vi "Create PublicEvents.vi"(5 "PublicEvents in":refnum<class "PublicEvents.lvclass">, 8 "error in (no error)":errorcluster, 11 "SMO":refnum<class "SMO.lvclass">) -> (0 "error out":errorcluster, 3 "PublicEvents":refnum<class "PublicEvents.lvclass">)   [LabVIEW 2013, in "PublicEvents.lvclass"]
uses:
  PublicEvents.lvclass
  SMO/SMO.lvclass
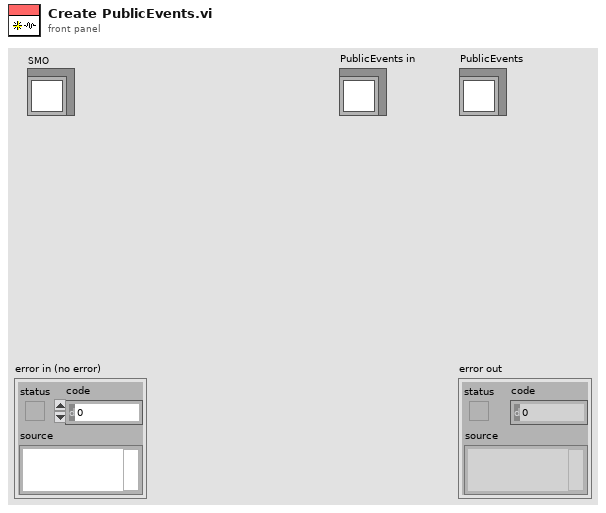
[diagram p1: front panel]
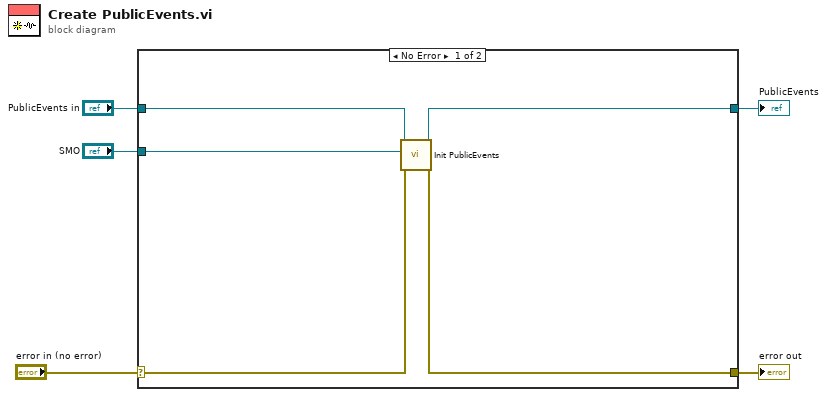
[diagram p0: block diagram]
diagram:
  n1 = case shown="No Error" "error in (no error)" {
    selector: "error in (no error)" -> [w8 w12]
    tunnel: [w7 w12] -> w4
    tunnel: [w9 w11] -> w3
    tunnel: "PublicEvents in" -> [w10 w11]
    tunnel: "SMO" -> [w6 _]
    frame No Error {
      n2 = call-dynamic "Init PublicEvents.vi"("error in (no error)"=w8, "SMO"=w6, "PublicEvents"=w10) -> ("error out"=w7:errorcluster, "PublicEvents"=w9:refnum<class "PublicEvents.lvclass">)  [unwired: 7 in]
    }
    frame Error {
    }
  }
  "error out" <- w4
  "PublicEvents" <- w3
